vi "ledmatrix.vi"() -> ()   [LabVIEW 2016]
uses:
  ledmatrix_default.ctl
  <vilib>/Instr/_visa.llb/VISA Configure Serial Port (Instr).vi
panel:
  out "error out":errorcluster
  in  "VISA resource name":refnum<visa-resource-name>="COM5"
  out "return count":u32
  in  "OK Button 2":bool
  in  "OK Button":bool
  in  "stop":bool
  out "String":string
  out "output array":u8[](array[numeric])
  in  "Array":T1
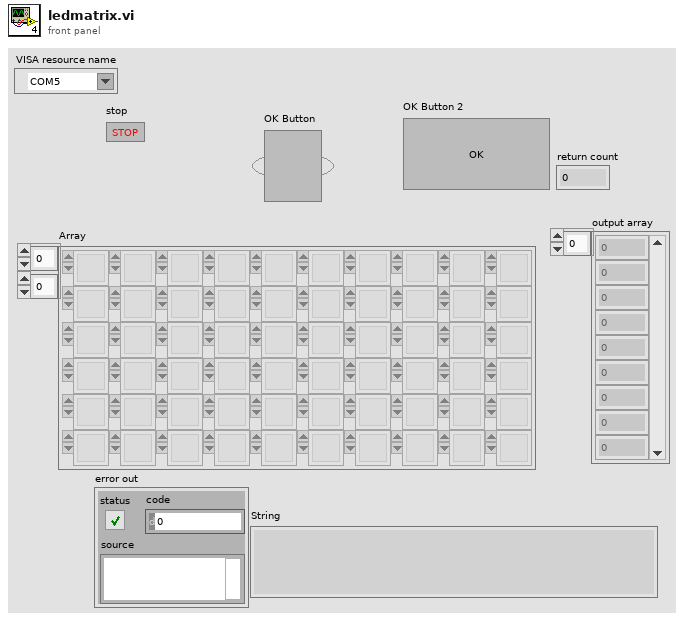
[diagram p1: front panel]
types:
  T1 = typedef "ledmatrix_default.ctl" = u8[][]
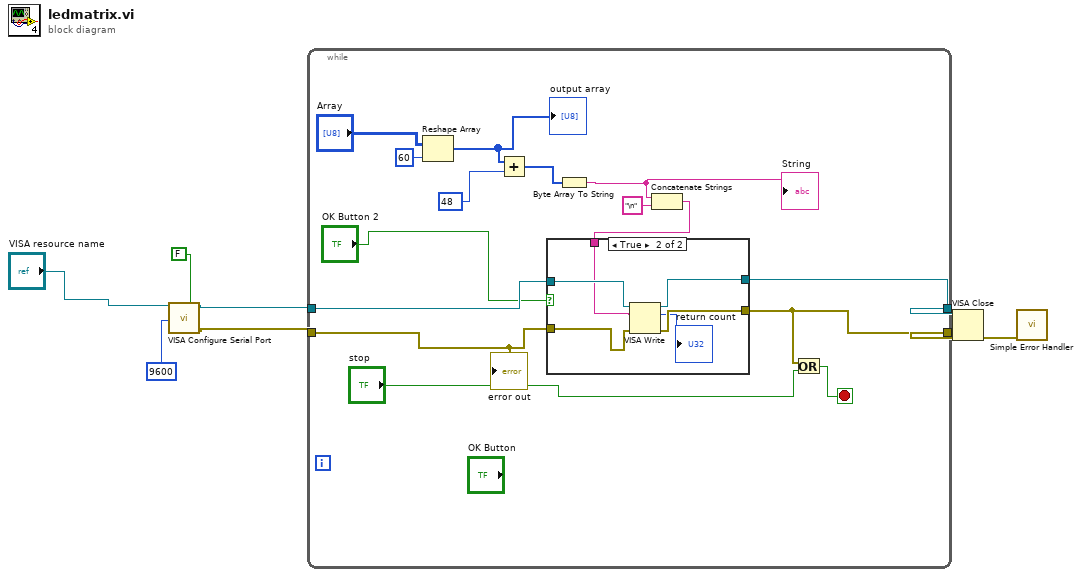
[diagram p0: block diagram]
diagram:
  n1 = call-poly "VISA Configure Serial Port"("VISA resource name"="VISA resource name", "Enable Termination\nChar (T)"=FALSE ("Enable Termination\nChar (T)"), "baud rate (9600)"=u32 9600) -> ("VISA resource name out"=w6:refnum<visa-resource-name>, "error out"=w5:errorcluster)  [unwired: 11 in]
  n2 = while {
    tunnel: w6 -> [w16]
    tunnel: w5 -> [w15]
    tunnel: [w13] -> w2
    tunnel: [w14] -> w3
    stop <- w17 stop-if-true
    n3 = Reshape Array("Array", 60 ("dimension size")) -> (w21:u8[])
    "output array" <- w21
    n4 = Add(x=w21, y=u8 48 ("dimension size")) -> (x+y=w23:u8[])
    n5 = Byte Array To String(unsigned byte array=w23) -> (string=w11:string)
    "String" <- w11
    n6 = Concatenate Strings(w11, "\n" ("string")) -> (w9:string)
    n7 = case shown="True" "OK Button 2" {
      tunnel: w9 -> [_ w30]
      tunnel: w16 -> [w25 w31]
      tunnel: w15 -> [w24 w29]
      tunnel: [w25 w27] -> w14
      tunnel: [w24 w28] -> w13
      frame False {
      }
      frame True {
        n8 = VISA Write(VISA resource name=w31, write buffer=w30, error in (no error)=w29) -> (VISA resource name out=w27:refnum<visa-resource-name>, return count=→"return count":u32, error out=w28:errorcluster)
      }
    }
    n9 = Or(x=w13, y="stop") -> (x .or. y?=w17:bool)
    "error out" <- w15
  }
  n10 = VISA Close(VISA resource name=w3, error in (no error)=w2) -> (error out=w1:errorcluster)
  n11 = call <vilib>:"Simple Error Handler.vi"("error in (no error)"=w1) -> ()  [unwired: 4 in, 5 out]
